vi "CANFrame2SensorValVI.vi"(1 "input":u8[](array[numeric])) -> (0 "output cluster":T1)   [LabVIEW 2021]
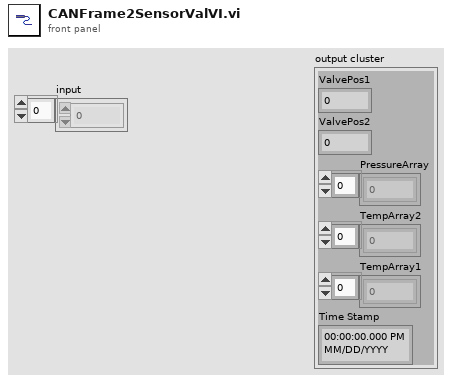
[diagram p1: front panel]
types:
  T1 = cluster{"ValvePos1":sgl, "ValvePos2":sgl, "PressureArray":sgl[], "TempArray2":sgl[], "TempArray1":sgl[], "Time Stamp":timestamp}
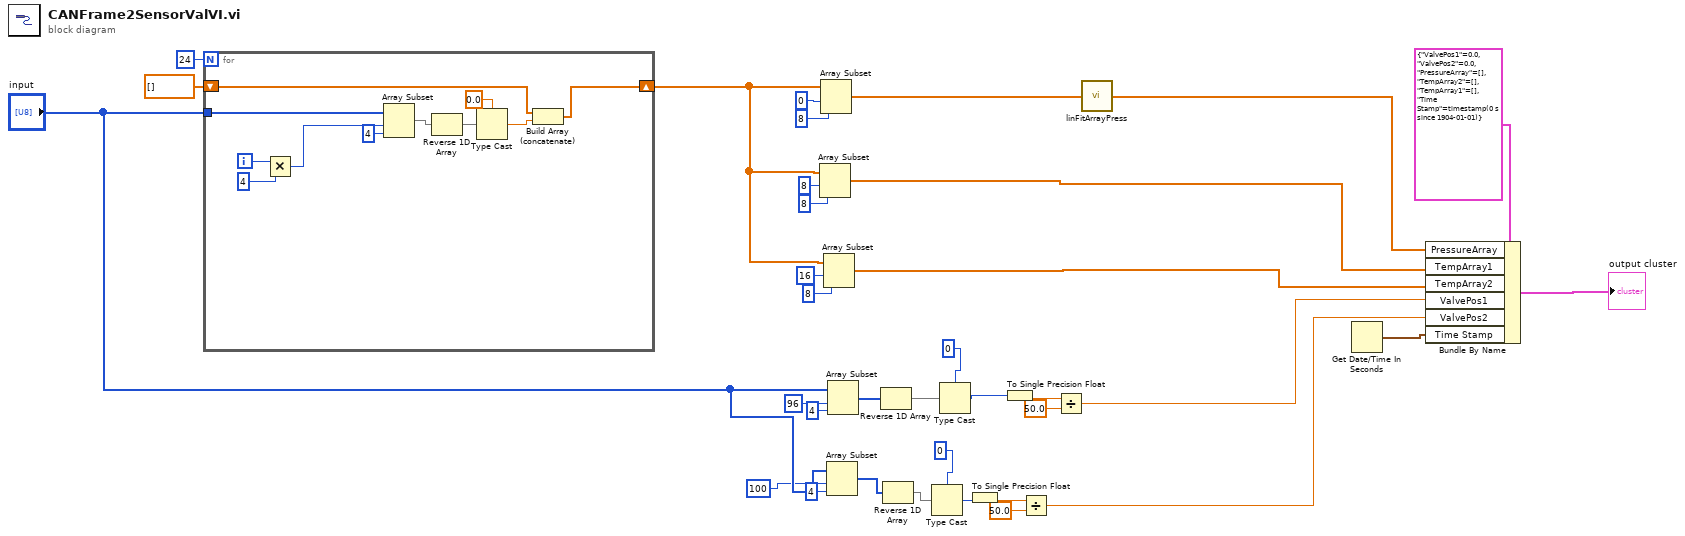
[diagram p0: block diagram]
diagram:
  n1 = for {
    N: 24 -> [_]
    tunnel: "input" -> [w44]
    shift-right: [w38] -> w33
    shift-left: sgl[] [] -> [w37]
    i -> [w46]
    n2 = Multiply(x=w46, y=4) -> (x*y=w43:i32)
    n3 = Array Subset(array=w44, index=w43, length=4) -> (w40:u8[])
    n4 = Reverse 1D Array(array=w40) -> (reversed array=w41:u8[])
    n5 = Type Cast(type=sgl 0.0, x=w41) -> (*(type *) &x=w39:sgl)
    n6 = Build Array (concatenate)(w37, w39) -> (w38:sgl[])
  }
  n7 = Array Subset(array=w33, index=8, length=8) -> (w11:sgl[])
  n8 = Array Subset(array=w33, index=0, length=8) -> (w4:sgl[])
  n9 = Array Subset(array=w33, index=16, length=8) -> (w10:sgl[])
  n10 = Array Subset(array="input", index=100, length=4) -> (w1:u8[])
  n11 = Array Subset(array="input", index=96, length=4) -> (w19:u8[])
  n12 = Reverse 1D Array(array=w19) -> (reversed array=w18:u8[])
  n13 = Reverse 1D Array(array=w1) -> (reversed array=w2:u8[])
  n14 = Type Cast(type=0, x=w2) -> (*(type *) &x=w12:i32)
  n15 = Type Cast(type=0, x=w18) -> (*(type *) &x=w17:i32)
  n16 = To Single Precision Float(number=w12) -> (single precision float=w14:sgl)
  n17 = To Single Precision Float(number=w17) -> (single precision float=w16:sgl)
  n18 = Divide(x=w14, y=sgl 50.0) -> (x/y=w8:sgl)
  n19 = Divide(x=w16, y=sgl 50.0) -> (x/y=w9:sgl)
  n20 = call "linFitArrayPress.vi"("volt"=w4) -> ("press"=w3:sgl[])
  n21 = Get Date/Time In Seconds() -> (seconds since 1Jan1904=w5:timestamp)
  n22 = Bundle By Name(cluster=T1 {"ValvePos1"=0.0, "ValvePos2"=0.0, "PressureArray"=[], "TempArray2"=[], "TempArray1"=[], "Time Stamp"=timestamp(0 s since 1904-01-01)} ("Cluster"), "PressureArray"=w3, "TempArray1"=w11, "TempArray2"=w10, "ValvePos1"=w9, "ValvePos2"=w8, "Time Stamp"=w5) -> (→"output cluster":T1)
